vi "InitMultipleDevices.vi"(4 "error in (no error)":errorcluster, 6 "msecDelayForDiscovery":i32, 7 "logging":bool) -> (0 "error out":errorcluster, 2 "DeviceKey List Out":string[](array[string]), 3 "CmdLib Out":refnum<k24>)   [LabVIEW 2013]
uses:
  C:/Users/Saffmanlab/Documents/git/CsPyController/labview/cesium_controller/PicoMotor/NewFocus8742/CmdLib.dll
  CmdLib.dll
panel:
  in  "deviceKeys":string[](array[string])
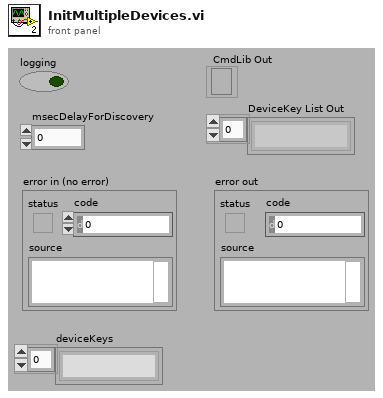
[diagram p1: front panel]
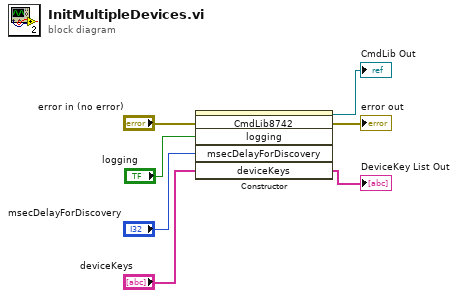
[diagram p0: block diagram]
diagram:
  n1 = constructor class="CmdLib8742"(error in="error in (no error)", "logging"="logging", "msecDelayForDiscovery"="msecDelayForDiscovery", "deviceKeys"="deviceKeys") -> (reference out=→"CmdLib Out":refnum<k24>, error out=→"error out":errorcluster, "deviceKeys"=→"DeviceKey List Out":string[])  [unwired: 2 in, 3 out]
